vi "Settings Dialog.vi"(8 "error in (no error)":errorcluster, 11 "Configuration in":T1={"Hardware Configuration"={"VGC50"={"serial settings"={"port"="", "baud rate"=115200}, "device information"={"type"="", "model number"="", "serial number"="", "firmware version"="", "hardware version"=""}, "gauges"=[], "VGC"=refnum, "Backing SP"={"mode"=0, "thresholds"={"lower"=0.0, "upper"=0.0}, "on"=FALSE}, "Chamber SP"={"mode"=1, "thresholds"={"lower"=0.0, "upper"=0.0}, "on"=FALSE}}, "PTC10"={"serial settings"={"port"="GPIB0::22::INSTR", "baud rate"=115200}, "PTC10 Info"={"Manufacturer"="", "Instrument"="", "Serial Number"="", "Firmware"=""}, "VISA resource name"="", "pwmloop"="define pwmloop(#t=0 while (1) {waitforsample if(#pwm=0){relays=0}else{if(#t<#pwm) {relays=1}else{relays=3}}#t+=1 if  (#t>99){#t=0} pause 0.2 s})", "onecycle"="define onecycle (pwm=100 run pwmloop 5A.PID.Setpoint=-130.0 5A.PID.input=3C while(#3C>-129.0){pause 0.2 s}pwm=-130 pause 10 min pwm=0  5A.PID.SetPoint=50.0 while(#3C<49.0){pause 0.2 s} pause 10 min kill pwmloop)", "control"="define control (#count=1 while (#count>=0) {onecycle pause 1 s #count-=1})", "Failsafe"="define Failsafe (while(1) {if (#Check <-20){relays=0 outputEnable Off}else{if(#Check>20){relays=0 outputEnable Off}} pause 1 s})", "ToAmbient"="define ToAmbient(if(#3C>25.0){pwm=100 run pwmloop while(#3C>#25.0){pause 0.5 s} pwm=0 kill pwmloop}else{#5A.PID.setpoint=20.0 while(#3C<15.0){pause 0.5 s} outputenable off})", "StartupCode"="system.display.Monitors Show", "LogChannels"=[], "Heater O/P Channel"="", " Control Input"="", "TAmbient"=20.0, "AmbientTolerance"=5.0, "TestCycleParameters"={"TAmb"=20.0, "HeaterTestTemp"=51.5, "HeaterTestDwell"=20, "HeaterTestDuration"=20, "MinOpTemp"=1.0, "MinOpDwell(min)"=1, "TestHeatingRate (deg/min)"=-131.5, "SurviveCycleParameters"={"MinSurviveTemp"=-131.5, "MinSurvive Dwell"=10, "MaxOpTemp"=50.0, "MaxOpDwell"=30, "ControlInput"=2, "ColdStandOff"=4.0, "HotStandoff"=5.0, "SteadyPWM"=20, "MaxCoolingRate (deg/min)"=3.75, "MaxHeatingRate (deg/min)"=2.5}}, "PID Params"={"P"=1.14, "I"=0.012, "D"=21.68}}}, "New Data Behavior"=enum."Replace", "Vacuum Graph config"={"Log/Lin"=FALSE, "Show Backing"=FALSE, "Show Chamber"=FALSE}} {"Hardware Configuration"."PTC10"."PID Params"."D" min=0.0; "Hardware Configuration"."PTC10"."PID Params"."I" min=0.0; "Hardware Configuration"."PTC10"."PID Params"."P" min=0.0; "Hardware Configuration"."PTC10"."TestCycleParameters"."SurviveCycleParameters"."SteadyPWM" min=0 max=100 step=1; "Hardware Configuration"."PTC10"."TestCycleParameters"."SurviveCycleParameters"."ControlInput" items=["3A", "3B", "3C", "3D", "4A", "4B", "4C", "4D"]; "Hardware Configuration"."PTC10"."serial settings"."baud rate" items=["9600"=9600, "19200"=19200, "38400"=38400, "57600"=57600, "115200"=115200]; "Hardware Configuration"."VGC50"."Chamber SP"."thresholds"."upper" format="%#_5p"; "Hardware Configuration"."VGC50"."Chamber SP"."thresholds"."lower" format="%#_5p"; "Hardware Configuration"."VGC50"."Chamber SP"."mode" items=["off", "on", "channel 1", "channel 2", "channel 3"]; "Hardware Configuration"."VGC50"."Backing SP"."thresholds"."upper" format="%#_5p"; "Hardware Configuration"."VGC50"."Backing SP"."thresholds"."lower" format="%#_5p"; "Hardware Configuration"."VGC50"."Backing SP"."mode" items=["off", "on", "channel 1", "channel 2", "channel 3"]; "Hardware Configuration"."VGC50"."gauges"."status" items=["data ok", "underrange", "overrange", "sensor error", "sensor off", "no sensor", "identification error", "error BPG, HPG, BCG"]; "Hardware Configuration"."VGC50"."gauges"."value" format="%#_4p"; "Hardware Configuration"."VGC50"."serial settings"."baud rate" items=["9600"=9600, "19200"=19200, "38400"=38400, "57600"=57600, "115200"=115200]}) -> (0 "error out":errorcluster, 2 "UI Refresh Needed?":bool, 3 "Configuration out":T1={"Hardware Configuration"={"VGC50"={"serial settings"={"port"="", "baud rate"=115200}, "device information"={"type"="", "model number"="", "serial number"="", "firmware version"="", "hardware version"=""}, "gauges"=[], "VGC"=refnum, "Backing SP"={"mode"=0, "thresholds"={"lower"=0.0, "upper"=0.0}, "on"=FALSE}, "Chamber SP"={"mode"=1, "thresholds"={"lower"=0.0, "upper"=0.0}, "on"=FALSE}}, "PTC10"={"serial settings"={"port"="GPIB0::22::INSTR", "baud rate"=115200}, "PTC10 Info"={"Manufacturer"="", "Instrument"="", "Serial Number"="", "Firmware"=""}, "VISA resource name"="", "pwmloop"="define pwmloop(#t=0 while (1) {waitforsample if(#pwm=0){relays=0}else{if(#t<#pwm) {relays=1}else{relays=3}}#t+=1 if  (#t>99){#t=0} pause 0.2 s})", "onecycle"="define onecycle (pwm=100 run pwmloop 5A.PID.Setpoint=-130.0 5A.PID.input=3C while(#3C>-129.0){pause 0.2 s}pwm=-130 pause 10 min pwm=0  5A.PID.SetPoint=50.0 while(#3C<49.0){pause 0.2 s} pause 10 min kill pwmloop)", "control"="define control (#count=1 while (#count>=0) {onecycle pause 1 s #count-=1})", "Failsafe"="define Failsafe (while(1) {if (#Check <-20){relays=0 outputEnable Off}else{if(#Check>20){relays=0 outputEnable Off}} pause 1 s})", "ToAmbient"="define ToAmbient(if(#3C>25.0){pwm=100 run pwmloop while(#3C>#25.0){pause 0.5 s} pwm=0 kill pwmloop}else{#5A.PID.setpoint=20.0 while(#3C<15.0){pause 0.5 s} outputenable off})", "StartupCode"="system.display.Monitors Show", "LogChannels"=[], "Heater O/P Channel"="", " Control Input"="", "TAmbient"=20.0, "AmbientTolerance"=5.0, "TestCycleParameters"={"TAmb"=20.0, "HeaterTestTemp"=51.5, "HeaterTestDwell"=20, "HeaterTestDuration"=20, "MinOpTemp"=1.0, "MinOpDwell(min)"=1, "TestHeatingRate (deg/min)"=-131.5, "SurviveCycleParameters"={"MinSurviveTemp"=-131.5, "MinSurvive Dwell"=10, "MaxOpTemp"=50.0, "MaxOpDwell"=30, "ControlInput"=2, "ColdStandOff"=4.0, "HotStandoff"=5.0, "SteadyPWM"=20, "MaxCoolingRate (deg/min)"=3.75, "MaxHeatingRate (deg/min)"=2.5}}, "PID Params"={"P"=1.14, "I"=0.012, "D"=21.68}}}, "New Data Behavior"=enum."Replace", "Vacuum Graph config"={"Log/Lin"=FALSE, "Show Backing"=FALSE, "Show Chamber"=FALSE}} {"Hardware Configuration"."PTC10"."PID Params"."D" min=0.0; "Hardware Configuration"."PTC10"."PID Params"."I" min=0.0; "Hardware Configuration"."PTC10"."PID Params"."P" min=0.0; "Hardware Configuration"."PTC10"."TestCycleParameters"."SurviveCycleParameters"."SteadyPWM" min=0 max=100 step=1; "Hardware Configuration"."PTC10"."TestCycleParameters"."SurviveCycleParameters"."ControlInput" items=["3A", "3B", "3C", "3D", "4A", "4B", "4C", "4D"]; "Hardware Configuration"."PTC10"."serial settings"."baud rate" items=["9600"=9600, "19200"=19200, "38400"=38400, "57600"=57600, "115200"=115200]; "Hardware Configuration"."VGC50"."Chamber SP"."thresholds"."upper" format="%#_5p"; "Hardware Configuration"."VGC50"."Chamber SP"."thresholds"."lower" format="%#_5p"; "Hardware Configuration"."VGC50"."Chamber SP"."mode" items=["off", "on", "channel 1", "channel 2", "channel 3"]; "Hardware Configuration"."VGC50"."Backing SP"."thresholds"."upper" format="%#_5p"; "Hardware Configuration"."VGC50"."Backing SP"."thresholds"."lower" format="%#_5p"; "Hardware Configuration"."VGC50"."Backing SP"."mode" items=["off", "on", "channel 1", "channel 2", "channel 3"]; "Hardware Configuration"."VGC50"."gauges"."status" items=["data ok", "underrange", "overrange", "sensor error", "sensor off", "no sensor", "identification error", "error BPG, HPG, BCG"]; "Hardware Configuration"."VGC50"."gauges"."value" format="%#_4p"; "Hardware Configuration"."VGC50"."serial settings"."baud rate" items=["9600"=9600, "19200"=19200, "38400"=38400, "57600"=57600, "115200"=115200]})   [LabVIEW 2024]
doc: "Dialog for selecting user specified settings."
uses:
  controls/User Specified Data.ctl
  <instrlib>/PL Inficon VGC/PL Inficon VGC.lvclass
  controls/HW Configuration.ctl
  controls/VGC50.ctl
  controls/SRS PTC10.ctl
  controls/TestCycleParams.ctl
  controls/SurviveCycleParams.ctl
  controls/ControlInput.ctl
  controls/PID Params.ctl
  controls/New Data Behavior.ctl
  controls/Vac Graph Config.ctl
panel:
  in  "New Data Behavior":u16(ring) items=["Replace", "Overlay", "Append"]
  in  "Cancel Button":bool
  in  "OK Button":bool
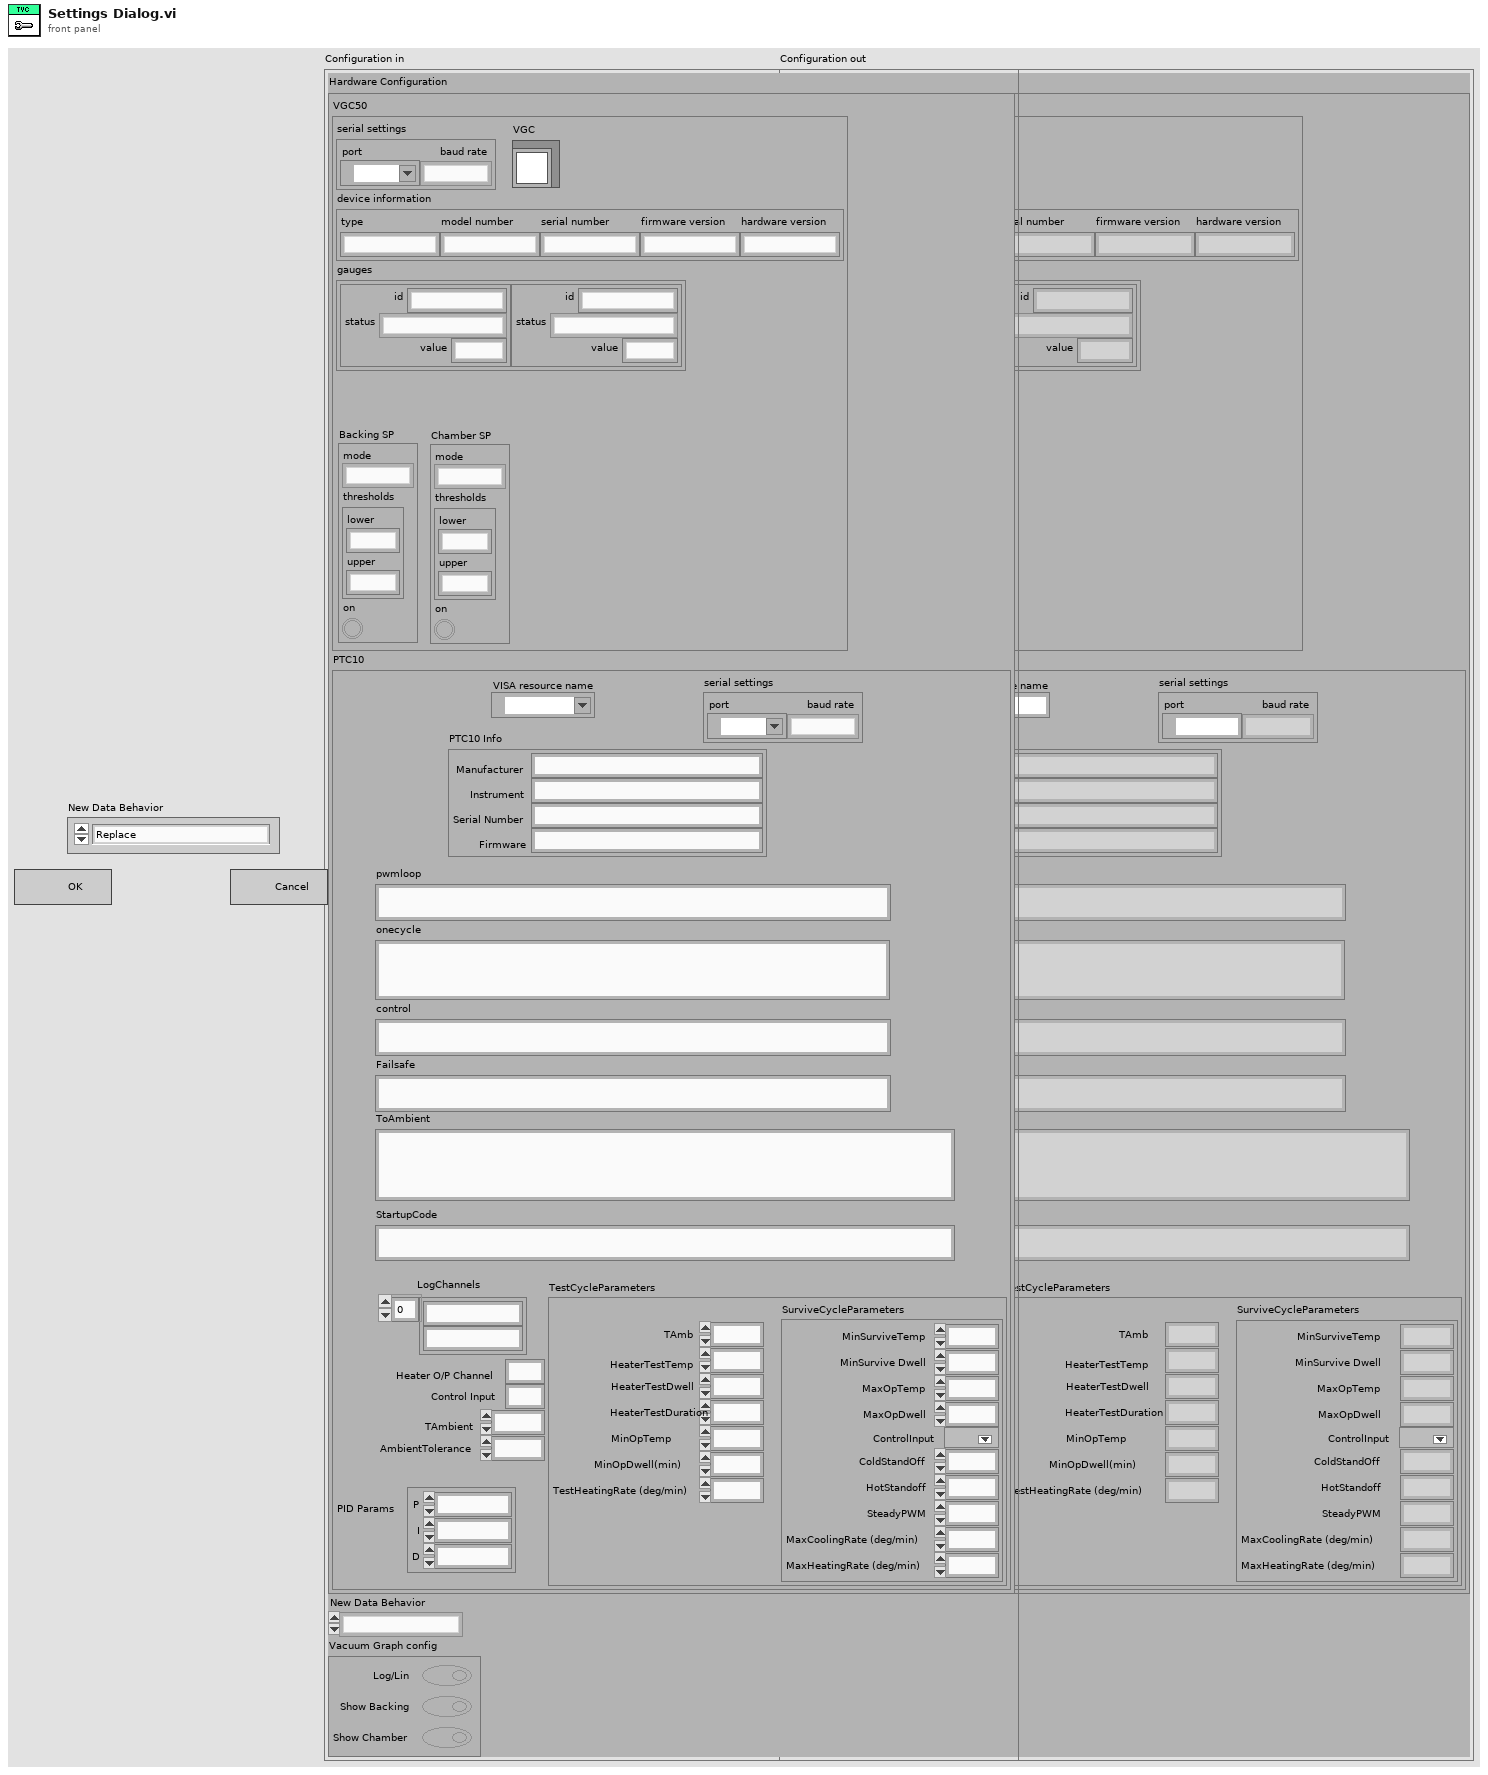
[diagram p1: front panel]
types:
  T1 = typedef "User Specified Data.ctl" = cluster{"Hardware Configuration":T2, "New Data Behavior":T9, "Vacuum Graph config":T10}
  T2 = typedef "HW Configuration.ctl" = cluster{"VGC50":T3, "PTC10":T4}
  T3 = typedef "VGC50.ctl" = cluster{"serial settings":cluster{"port":refnum<visa-resource-name>, "baud rate":u32}, "device information":cluster{"type":string, "model number":string, "serial number":string, "firmware version":string, "hardware version":string}, "gauges":cluster{"id":string, "status":u16, "value":dbl}[], "VGC":refnum<class "PL Inficon VGC.lvclass">, "Backing SP":cluster{"mode":u16, "thresholds":cluster{"lower":dbl, "upper":dbl}, "on":bool}, "Chamber SP":cluster{"mode":u16, "thresholds":cluster{"lower":dbl, "upper":dbl}, "on":bool}}
  T4 = typedef "SRS PTC10.ctl" = cluster{"serial settings":cluster{"port":refnum<visa-resource-name>, "baud rate":u32}, "PTC10 Info":cluster{"Manufacturer":string, "Instrument":string, "Serial Number":string, "Firmware":string}, "VISA resource name":refnum<visa-resource-name>, "pwmloop":string, "onecycle":string, "control":string, "Failsafe":string, "ToAmbient":string, "StartupCode":string, "LogChannels":string[], "Heater O/P Channel":string, " Control Input":string, "TAmbient":dbl, "AmbientTolerance":dbl, "TestCycleParameters":T5, "PID Params":T8}
  T5 = typedef "TestCycleParams.ctl" = cluster{"TAmb":dbl, "HeaterTestTemp":dbl, "HeaterTestDwell":i32, "HeaterTestDuration":i32, "MinOpTemp":dbl, "MinOpDwell(min)":i32, "TestHeatingRate (deg/min)":dbl, "SurviveCycleParameters":T6}
  T6 = typedef "SurviveCycleParams.ctl" = cluster{"MinSurviveTemp":dbl, "MinSurvive Dwell":i32, "MaxOpTemp":dbl, "MaxOpDwell":i32, "ControlInput":T7, "ColdStandOff":dbl, "HotStandoff":dbl, "SteadyPWM":i32, "MaxCoolingRate (deg/min)":dbl, "MaxHeatingRate (deg/min)":dbl}
  T7 = typedef "ControlInput.ctl" = u16
  T8 = typedef "PID Params.ctl" = cluster{"P":dbl, "I":dbl, "D":dbl}
  T9 = typedef "New Data Behavior.ctl" = enum16{"Replace", "Overlay", "Append"}
  T10 = typedef "Vac Graph Config.ctl" = cluster{"Log/Lin":bool, "Show Backing":bool, "Show Chamber":bool}
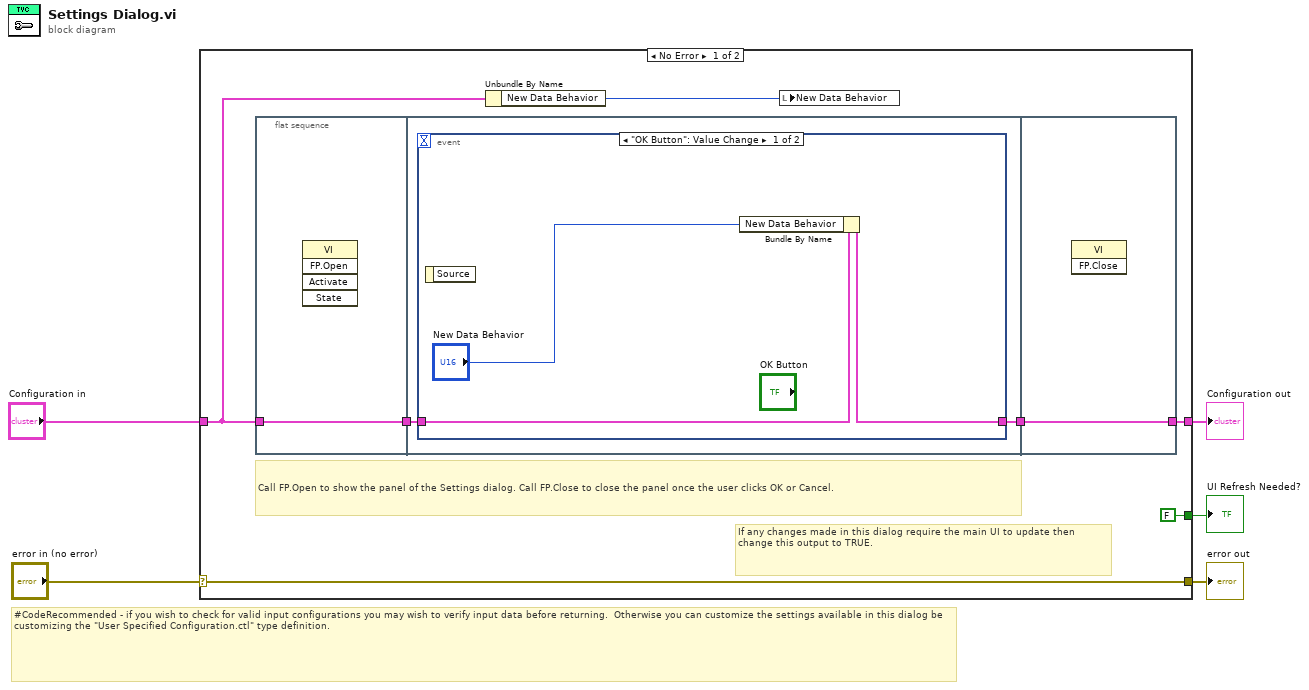
[diagram p0: block diagram]
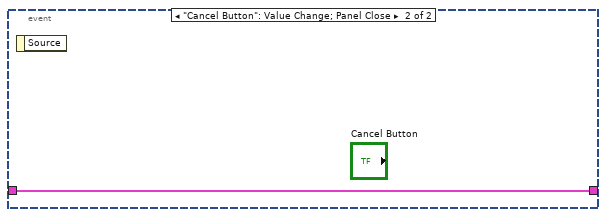
[diagram p2: hidden frame]
diagram:
  # "#CodeRecommended - if you wish to check for valid input configurations you may wish to verify input data before returning.  Otherwise you can customize the settings available in this dialog be customizing the \"User Specified Configuration.ctl\" type definition."
  n1 = case shown="No Error" "error in (no error)" {
    selector: "error in (no error)" -> [w12 w22]
    tunnel: [w12 w22] -> w4
    tunnel: "Configuration in" -> [w9 w21]
    tunnel: [w11 w21] -> w2
    tunnel: [FALSE ("UI Refresh Needed?") _] -> w1
    frame No Error {
      # "Call FP.Open to show the panel of the Settings dialog. Call FP.Close to close the panel once the user clicks OK or Cancel."
      # "If any changes made in this dialog require the main UI to update then change this output to TRUE."
      n2 = flat-sequence {
        tunnel: w9 -> [w13]
        tunnel: [w13] -> w7
        tunnel: w7 -> [w14]
        tunnel: [w15] -> w6
        tunnel: [w20] -> w11
        tunnel: w6 -> [w20]
        frame #0 {
          n3 = invoke class="VI" method="FP.Open"() -> ()  [unwired: 5 in, 5 out]
        }
        frame #1 {
          n4 = event shown="[0] \"OK Button\": Value Change" {
            selector: _ -> [_ _]
            dyn-events: _ -> [_ _]
            timeout: _ -> [_ _]
            tunnel: [w17 w19] -> w15
            tunnel: w14 -> [w18 w19]
            event "OK Button": Value Change {
              n5 = event-data() -> ()  [unwired: 1 in, 1 out]
              n6 = Bundle By Name(cluster=w18, "New Data Behavior"="New Data Behavior") -> (w17:T1)
            }
            event "Cancel Button": Value Change; Panel Close {
              n7 = event-data() -> ()  [unwired: 1 in, 1 out]
            }
          }
        }
        frame #2 {
          n8 = invoke class="VI" method="FP.Close"() -> ()  [unwired: 3 in, 3 out]
        }
      }
      n9 = Unbundle By Name(w9) -> ("New Data Behavior"=w8:T9)
      n10 = local write "New Data Behavior"(w8) -> ()
    }
    frame Error {
    }
  }
  "UI Refresh Needed?" <- w1
  "error out" <- w4
  "Configuration out" <- w2
